vi "Add Comment.vi"(9 "Max width (60)":i32=60, 10 "Comment":string="This is a really really really long sentence that should have to wrap to multiple lines.\n\nA new line!", 11 "String in":string) -> (3 "String out":string)   [LabVIEW 2013, in "C Header Generator.lvlib"]
uses:
  C Header Generator.lvlib
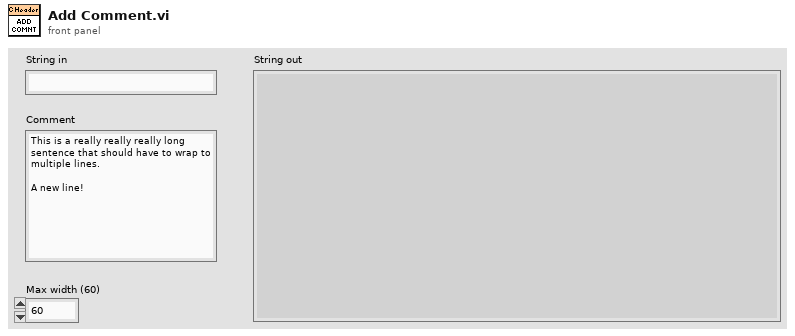
[diagram p1: front panel]
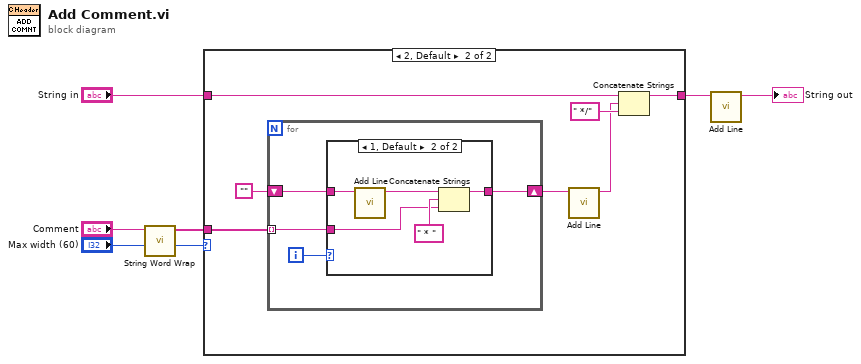
[diagram p0: block diagram]
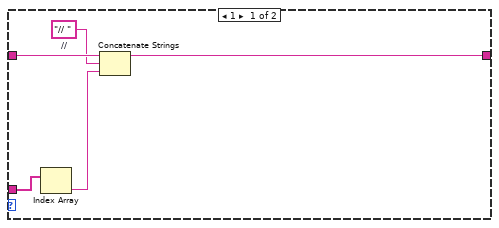
[diagram p2: hidden frame]
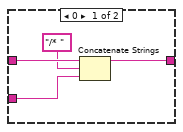
[diagram p3: hidden frame]
diagram:
  n1 = call "String Word Wrap.vi"("Max width (60)"="Max width (60)", "String in"="Comment") -> ("Number of lines"=w3:i32, "Wrapped lines"=w4:string[])  [unwired: 8 in]
  n2 = case shown="2, Default" w3 {
    tunnel: "String in" -> [w12 w16]
    tunnel: [w11 w15] -> w7
    tunnel: w4 -> [w9 w13]
    frame 1 {
      w10 = "// "  # //
      n3 = Index Array(array=w9) -> (element=w8:string)  [unwired: 1 in]
      n4 = Concatenate Strings(w12, w10, w8) -> (w11:string)
    }
    frame 2, Default {
      n5 = for {
        shift-right: [w23] -> w17
        shift-left: "" -> [w22]
        tunnel: w13 -> [w20] mode=indexing
        i -> [w21]
        n6 = case shown="1, Default" w21 {
          tunnel: w22 -> [w26 w30]
          tunnel: [w27 w32] -> w23
          tunnel: w20 -> [w24 w28]
          frame 0 {
            n7 = Concatenate Strings(w26, "/* ", w24) -> (w27:string)
          }
          frame 1, Default {
            n8 = call "Add Line.vi"("String in"=w30) -> ("String out"=w29:string)  [unwired: 10 in]
            n9 = Concatenate Strings(w29, " * ", w28) -> (w32:string)
          }
        }
      }
      n10 = call "Add Line.vi"("String in"=w17) -> ("String out"=w18:string)  [unwired: 10 in]
      n11 = Concatenate Strings(w16, w18, " */" ("string")) -> (w15:string)
    }
  }
  n12 = call "Add Line.vi"("String in"=w7) -> ("String out"=→"String out":string)  [unwired: 10 in]
